vi "Distance(single).vi"(1 "D2":dbl format="%.2f", 2 "D1":dbl format="%.2f") -> (0 "DT":dbl format="%.2f")   [LabVIEW 2011]
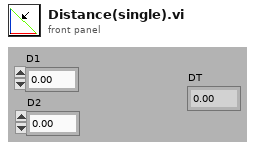
[diagram p1: front panel]
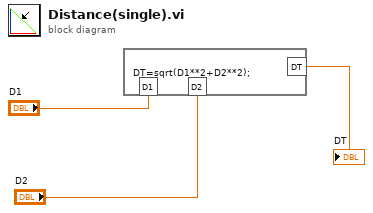
[diagram p0: block diagram]
diagram:
  n1 = formula code="DT=sqrt(D1**2+D2**2);"("D1"="D1", "D2"="D2") -> ("DT"=→"DT":dbl)
